vi "LCD.vi"(11 "String":string) -> ()   [LabVIEW 2017]
uses:
  <vilib>/myRIO/Instrument Drivers/Onboard IO/UART/typedef/VISA Configuration.ctl
  <vilib>/Instr/_visa.llb/VISA Configure Serial Port (Instr).vi
  <vilib>/myRIO/Express VI/Onboard IO/UART/UART Express VI.xnode
  <vilib>/myRIO/Instrument Drivers/Onboard IO/UART/UART.lvlib
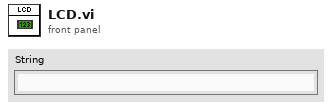
[diagram p1: front panel]
types:
  T1 = typedef "UART.lvlib/VISA Configuration.ctl" = cluster{"baud rate (9600)":u32, "data bits (8)":u16, "parity (0:none)":enum16{"None", "Odd", "Even", "Mark", "Space"}, "stop bits (10: 1 bit)":u16, "flow control (0:none)":u16, "termination char\n(0xA = '\\n' = LF) ":u8, "Enable Termination\nChar (T)":bool, "timeout (10sec)":u32}
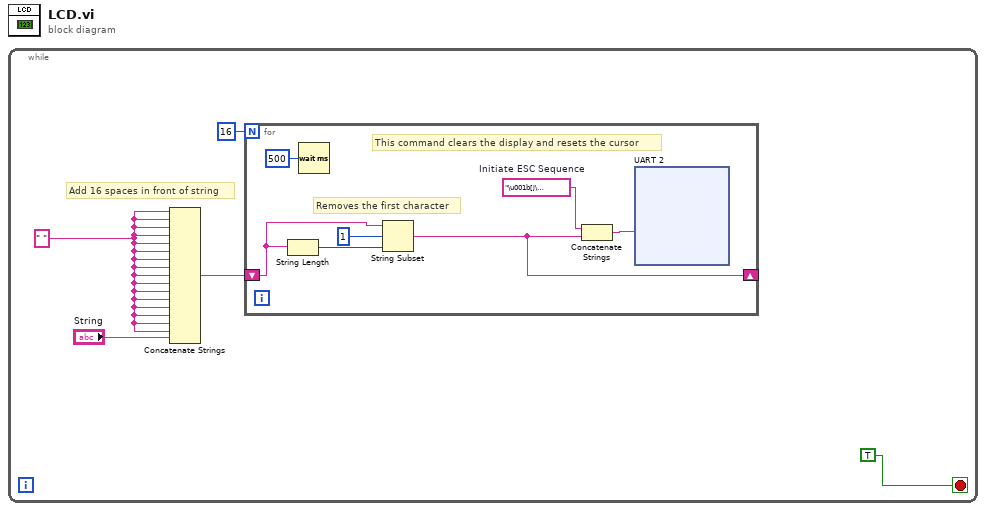
[diagram p0: block diagram]
diagram:
  n1 = while {
    stop <- TRUE stop-if-true
    w4 = " "
    # "Add 16 spaces in front of string"
    n2 = Concatenate Strings(w4, w4, w4, w4, w4, w4, w4, w4, w4, w4, w4, w4, w4, w4, w4, w4, "String") -> (w3:string)
    n3 = for {
      N: 16 -> [_]
      shift-right: [w7] -> _
      shift-left: w3 -> [w12]
      w8 = "\u001b[j\u001b[0h"  # Initiate ESC Sequence
      # "This command clears the display and resets the cursor"
      # "Removes the first character"
      n4 = String Length(string=w12) -> (length=w11:i32)
      n5 = Wait (ms)(milliseconds to wait=u32 500) -> ()  [unwired: 1 out]
      n6 = String Subset(string=w12, offset (0)=1, length (rest)=w11) -> (substring=w7:string)
      n7 = Concatenate Strings(w8, w7) -> (w9:string)
      n8 = xnode "UART 2"("Characters to Write"=w9) -> ()  [unwired: 1 in, 2 out]
    }
  }
